vi "TCP Build Error.vi"(1 "Error":string, 2 "error in (no error)":errorcluster, 3 "code":i32=7104) -> (0 "error out":errorcluster)   [LabVIEW 2018]
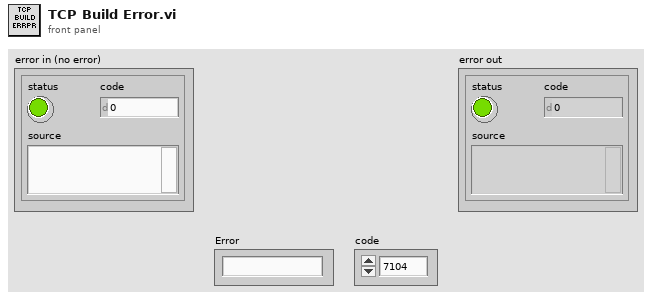
[diagram p1: front panel]
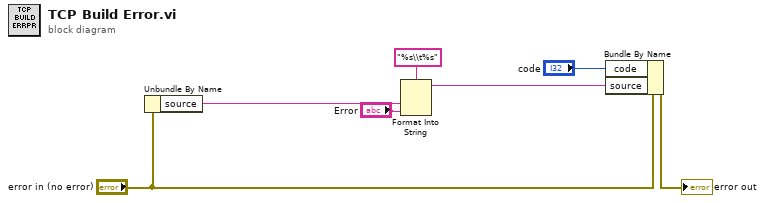
[diagram p0: block diagram]
diagram:
  n1 = Unbundle By Name("error in (no error)") -> ("source"=w3:string)
  n2 = Format Into String(format string="%s\\t%s", w3, "Error") -> (resulting string=w2:string)  [unwired: 2 in, 1 out]
  n3 = Bundle By Name(cluster="error in (no error)", "code"="code", "source"=w2) -> (→"error out":errorcluster)
